vi "HEWH Check Flag Modifier.vi"(8 "Error In":errorcluster, 9 "Terminate Input":bool, 10 "Station ID":T1, 11 "Cluster":T2 {"Time" format="%<%H:%M:%S>t"}) -> (0 "Error Out":errorcluster, 2 "Message Adder":string, 3 "Terminate Output":bool)   [LabVIEW 2016]
uses:
  Type Definitions/PRAT Test.ctl
  Utility/Save File/File Setup (Public)/Type Definition/Save File HEWH Heating Control Mode.ctl
  Type Definitions/Terminate Draw Conditions.ctl
  Type Definitions/HEWH Start Conditions.ctl
  Type Definitions/Check Special Condtions.ctl
  Type Definitions/HEWH Special Condition Check.ctl
  Type Definitions/HEWH Draw Flag ENUM.ctl
  Custom Instrument Control/MW100/Type Definitions/Station ID Selector.ctl
  Utility/Type Definitions/UTILITY Notifier.ctl
  Utility/Save File/File Setup.lvlib
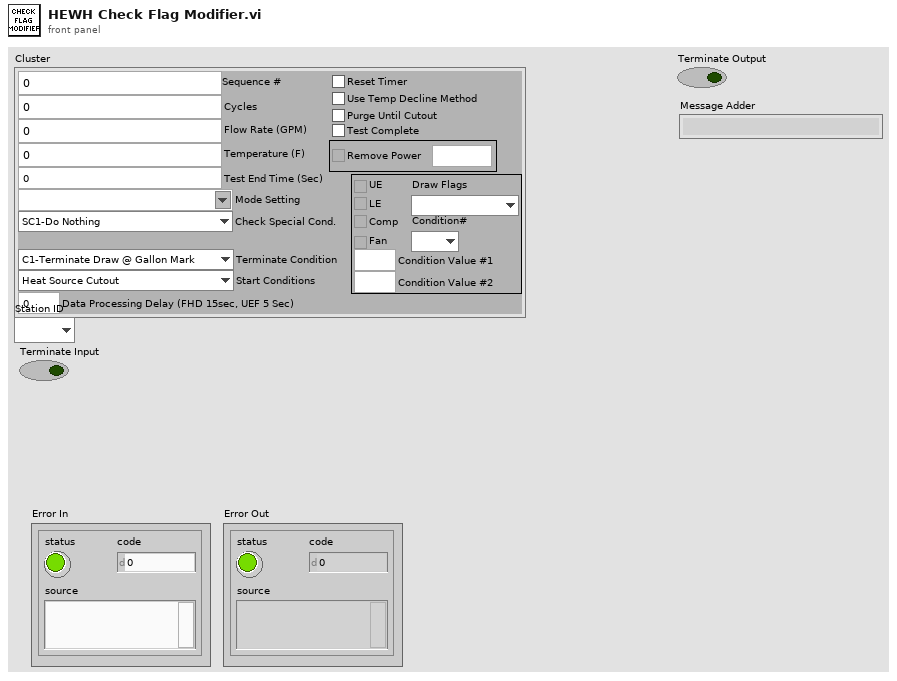
[diagram p1: front panel]
types:
  T1 = typedef "Station ID Selector.ctl" = enum16{"", "A", "B", "C", "D", "Global"}
  T2 = typedef "PRAT Test.ctl" = cluster{"Sequence #":dbl, "Cycles":i32, "Mode Setting":T3, "Flow Rate (GPM)":dbl, "Temperature (F)":dbl, "Reset Timer":bool, "Use Temp Decline Method":bool, "Terminate Condition":T4, "Condition Value #1":dbl, "UE":bool, "LE":bool, "Comp":bool, "Fan":bool, "Test End Time (Sec)":dbl, "Purge Until Cutout":bool, "Start Conditions":T5, "Condition Value #2":dbl, "Remove Power":bool, "Time":dbl, "Check Special Cond.":T6, "Condition#":T7, "Draw Flags":T8, "Data Processing Delay (FHD 15sec, UEF 5 Sec)":dbl, "Test Complete":bool}
  T3 = typedef "File Setup.lvlib/Save File HEWH Heating Control Mode.ctl" = string
  T4 = typedef "Terminate Draw Conditions.ctl" = enum16{"C1-Terminate Draw @ Gallon Mark", "C2-Special Last Draw (HU Test)", "C3-RTD Out <=", "C4-Mean Tank Temp <=", "C5-Decrease RTD Out (Deg F)", "C6-Time (Seconds)", "C7-Until Any Heat Source", "C8-Specific Heat Source", "C9-Do Nothing"}
  T5 = typedef "HEWH Start Conditions.ctl" = enum16{"Heat Source Cutout", "At Time (Seconds)", "Every X (Seconds)", "T2 >= X° Below Setpoint", "Seconds From Complete", "Wait for LE & Comp Cutout", "Wait for Comp Cutout", "Wait for LE Cutout", "Wait for UE Cutout"}
  T6 = typedef "Check Special Condtions.ctl" = enum16{"SC1-Do Nothing", "SC2-Check Heat Source (On-C2/Off-C1)", "SC3-Check Skip Condition", "SC4-Check Heat Source ON/Fail"}
  T7 = typedef "HEWH Special Condition Check.ctl" = enum16{"N/A", "C1", "C2", "Reset/Fail", "Skip Draw Sequence"}
  T8 = typedef "HEWH Draw Flag ENUM.ctl" = enum16{"N/A", "None(0)", "Sml(1)", "Med(2)", "SmlMed(3)", "Lrg(4)", "SmlLrg(5)", "MedLrg(6)", "SmlMedLrg(7)"}
  T9 = typedef "UTILITY Notifier.ctl" = enum16{"Set", "Read", "Release Ref"}
  T10 = typedef "GEA2 Commands WaterHeater GEA2 Data.ctl" = cluster{"GEA2 Label Array":string[], "PID_PARAMETERS":string[][], "SUPPORTED_MODES":string[][], "Button Status":T11, "Status Query":T12, "Service Error Codes":T13, "HEM_KWH_DATA":string[][], "OTHER_FAULT_COUNTS":string[][], "GEA2 Raw Message":string, "Hyperterminal Data":cluster{"Source":u8, "Destination":u8, "Command":u8, "Length":u8, "CRC":u16, "UE - state (1/0 on off)":u8, "LE - state (1/0 on off)":u8, "Comp - state (1/0 on off)":u8, "Fan  - state (1/0 on off)":u8, "Setpoint Deg F":i32, "T2(TankSensor)":dbl, "T3A(EvapIn)":dbl, "T3B(EvapOut)":dbl, "T4(CompressorDischarge)":dbl, "T5(Ambient)":dbl, "Current":dbl, "Voltage (Volts)":u16, "EEV Position (0-480)":u16, "Reason for last heating cycle termination":u16, "Reason Data word 1":string, "Reason Data word 2":string, "Reason Data word 3":string, "Reason Data word 4":string, "SW Debug Data":string, "Flow Events (Bit Encoded)":u16, "Heating Control Mode":u16}, "Extra Data":cluster{"Water Capacity (Gallons)":u32, "Max Vacation Duration Days":u32, "Min Vacation Duration Days":u32, "Max Set Point (Deg F)":u32, "Min Set Point (Deg F)":u32, "T5 Resistance":u32, "T4 Resistance":u32, "T3B Resistance":u32, "T2 Resistance":u32, "STD_ELEC_RANGE":string, "SS_FAULT_COUNTS":string, "SERIAL_NUMBER":string, "READ_PERSONALITY":u8, "RQST_OVERRIDE_STATUS":string, "MODEL_SELECT_AD_VALUE":u32, "MODEL NUMBER":string, "IDLB_RESISTANCE":u32, "DSM Override Status":string, "RQST_DATA_FROM_Memory":string, "RQST_DATA_FROM_DATA_FLASH":string, "RQST_CURRENT_PID_SH_TARGET":u16, "Unit System Mode":string}}
  T11 = typedef "GEA2 Commands Button Status.ctl" = cluster{"Switch 1":bool, "Switch 2":bool, "Switch 3":bool, "Switch 4":bool, "Switch 5":bool, "Switch 6":bool, "Switch 7":bool, "Switch 8":bool, "Switch 9":bool, "Switch 10":bool, "Switch 11":bool, "Switch 12":bool, "Switch 13":bool, "Switch 14":bool, "Switch 15":bool, "Switch 16":bool}
  T12 = typedef "GEA2 Commands Status Query.ctl" = cluster{"Days Remaining (For Std Electric and Vacation)":u8, "Unit Status":string, "Current Tank Temp in Deg F":u8, "Current Setpoint in Deg F":u8, "Filter Status (% used)":u8, "Fallback Status (Fallback heating mode)":string, "Fallback Temp":u8, "\"Set Mode\" Selection":string}
  T13 = typedef "GEA2 Commands Service Error Codes.ctl" = cluster{"Reserved":bool, "Reserved 1":bool, "Reserved 2":bool, "Reserved 3":bool, "Reserved 4":bool, "Reserved 5":bool, "Reserved 6":bool, "Reserved 7":bool, "DataFlash Fail Status":bool, "Stuck Key Fail Status":bool, "Dry Tank Fail Status":bool, "Miswire Fail Status":bool, "Reserved 8":bool, "Reserved 9":bool, "Reserved 10":bool, "Reserved 11":bool, "UE Fail Status":bool, "LE Fail Status":bool, "Filter Fail Status":bool, "T3A Fail Status":bool, "T3B Fail Status":bool, "T4 Fail Status":bool, "T5 Fail Status":bool, "T2 Fail Status":bool, "SS Cond A Status":bool, "SS Cond B Status":bool, "SS Cond C Status":bool, "SS Cond D Status":bool, "SS Cond E Status":bool, "SS Cond F Status":bool, "SS Fan Status":bool, "CMP Fail Status":bool}
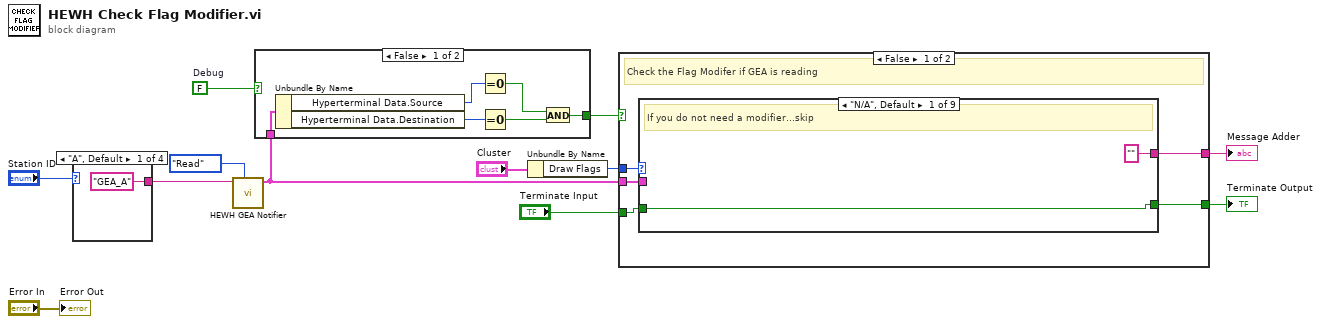
[diagram p0: block diagram]
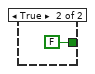
[diagram p2: hidden frame]
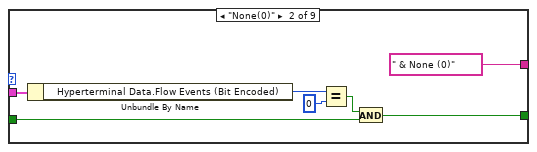
[diagram p3: hidden frame]
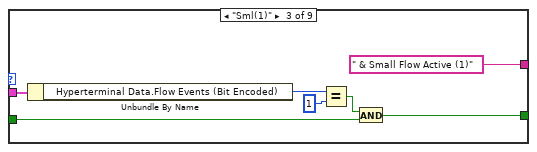
[diagram p4: hidden frame]
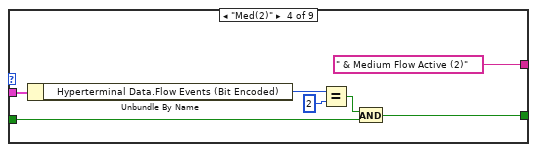
[diagram p5: hidden frame]
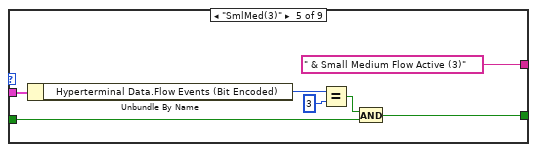
[diagram p6: hidden frame]
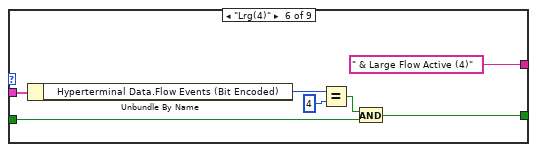
[diagram p7: hidden frame]
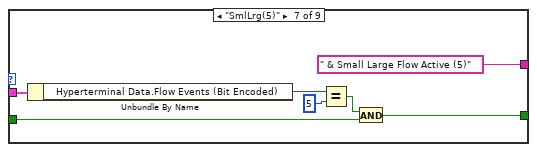
[diagram p8: hidden frame]
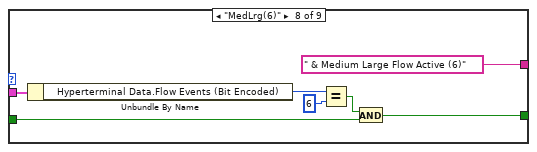
[diagram p9: hidden frame]
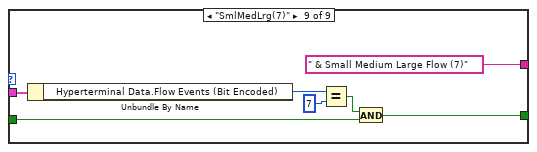
[diagram p10: hidden frame]
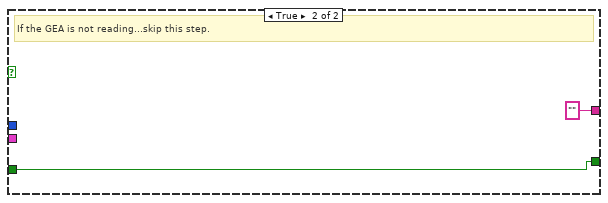
[diagram p11: hidden frame]
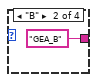
[diagram p12: hidden frame]
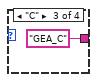
[diagram p13: hidden frame]
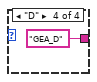
[diagram p14: hidden frame]
diagram:
  w1 = FALSE  # Debug
  n1 = case shown="\"A\", Default" "Station ID" {
    tunnel: ["GEA_A" ("name (unnamed)") "GEA_B" ("name (unnamed)") "GEA_C" ("name (unnamed)") "GEA_D" ("name (unnamed)")] -> w11
    frame "A", Default {
    }
    frame "B" {
    }
    frame "C" {
    }
    frame "D" {
    }
  }
  n2 = call "HEWH GEA Notifier.vi"("Status"=UTILITY_Notifier."Read", "name (unnamed)"=w11) -> ("latest notification"=w4:T10)  [unwired: 8 in, 1 out]
  n3 = case shown="False" w1 {
    tunnel: w4 -> [w22 _]
    tunnel: [w17 FALSE] -> w3
    frame False {
      n4 = Unbundle By Name(w22) -> ("Hyperterminal Data.Source"=w19:u8, "Hyperterminal Data.Destination"=w18:u8)
      n5 = Equal To 0?(x=w19) -> (x = 0?=w21:bool)
      n6 = Equal To 0?(x=w18) -> (x = 0?=w20:bool)
      n7 = And(x=w21, y=w20) -> (x .and. y?=w17:bool)
    }
    frame True {
    }
  }
  n8 = Unbundle By Name("Cluster") -> ("Draw Flags"=w7:T8)
  n9 = case shown="False" w3 {
    tunnel: w7 -> [w28 _]
    tunnel: "Terminate Input" -> [w27 w88]
    tunnel: [w26 w88] -> w5
    tunnel: w4 -> [w25 _]
    tunnel: [w24 ""] -> w2
    frame False {
      # "Check the Flag Modifer if GEA is reading"
      n10 = case shown="\"N/A\", Default" w28 {
        tunnel: w27 -> [w30 w33 w40 w48 w54 w61 w68 w74 w82]
        tunnel: [w30 w32 w39 w47 w53 w60 w67 w75 w81] -> w26
        tunnel: w25 -> [_ w37 w42 w46 w55 w62 w70 w76 w83]
        tunnel: ["" " & None (0)" " & Small Flow Active (1)" " & Medium Flow Active (2)" " & Small Medium Flow Active (3)" " & Large Flow Active (4)" " & Small Large Flow Active (5)" " & Medium Large Flow Active (6)" " & Small Medium Large Flow (7)"] -> w24
        frame "N/A", Default {
          # "If you do not need a modifier...skip"
        }
        frame "None(0)" {
          n11 = Unbundle By Name(w37) -> ("Hyperterminal Data.Flow Events (Bit Encoded)"=w36:u16)
          n12 = Equal?(x=w36, y=u16 0) -> (x = y?=w34:bool)
          n13 = And(x=w34, y=w33) -> (x .and. y?=w32:bool)
        }
        frame "Sml(1)" {
          n14 = Unbundle By Name(w42) -> ("Hyperterminal Data.Flow Events (Bit Encoded)"=w44:u16)
          n15 = Equal?(x=w44, y=u16 1) -> (x = y?=w41:bool)
          n16 = And(x=w41, y=w40) -> (x .and. y?=w39:bool)
        }
        frame "Med(2)" {
          n17 = Unbundle By Name(w46) -> ("Hyperterminal Data.Flow Events (Bit Encoded)"=w51:u16)
          n18 = Equal?(x=w51, y=u16 2) -> (x = y?=w49:bool)
          n19 = And(x=w49, y=w48) -> (x .and. y?=w47:bool)
        }
        frame "SmlMed(3)" {
          n20 = Unbundle By Name(w55) -> ("Hyperterminal Data.Flow Events (Bit Encoded)"=w58:u16)
          n21 = Equal?(x=w58, y=u16 3) -> (x = y?=w56:bool)
          n22 = And(x=w56, y=w54) -> (x .and. y?=w53:bool)
        }
        frame "Lrg(4)" {
          n23 = Unbundle By Name(w62) -> ("Hyperterminal Data.Flow Events (Bit Encoded)"=w65:u16)
          n24 = Equal?(x=w65, y=u16 4) -> (x = y?=w63:bool)
          n25 = And(x=w63, y=w61) -> (x .and. y?=w60:bool)
        }
        frame "SmlLrg(5)" {
          n26 = Unbundle By Name(w70) -> ("Hyperterminal Data.Flow Events (Bit Encoded)"=w72:u16)
          n27 = Equal?(x=w72, y=u16 5) -> (x = y?=w69:bool)
          n28 = And(x=w69, y=w68) -> (x .and. y?=w67:bool)
        }
        frame "MedLrg(6)" {
          n29 = Unbundle By Name(w76) -> ("Hyperterminal Data.Flow Events (Bit Encoded)"=w79:u16)
          n30 = Equal?(x=w79, y=u16 6) -> (x = y?=w77:bool)
          n31 = And(x=w77, y=w74) -> (x .and. y?=w75:bool)
        }
        frame "SmlMedLrg(7)" {
          n32 = Unbundle By Name(w83) -> ("Hyperterminal Data.Flow Events (Bit Encoded)"=w86:u16)
          n33 = Equal?(x=w86, y=u16 7) -> (x = y?=w84:bool)
          n34 = And(x=w84, y=w82) -> (x .and. y?=w81:bool)
        }
      }
    }
    frame True {
      # "If the GEA is not reading...skip this step."
    }
  }
  "Terminate Output" <- w5
  "Message Adder" <- w2
  "Error Out" <- "Error In"
